vi "Configure Time Tagging.vi"(7 "Virtual Memory Unit in":refnum<class "Virtual Memory Unit.lvclass">, 8 "error in (no error)":errorcluster, 11 "Bus Monitor in":refnum<class "Bus Monitor.lvclass">) -> (0 "error out":errorcluster, 3 "Bus Monitor out":refnum<class "Bus Monitor.lvclass">, 5 "Virtual Memory Unit out":refnum<class "Virtual Memory Unit.lvclass">)   [LabVIEW 2016, in "BCI-1553 API.lvlib" / "Bus Monitor.lvclass"]
uses:
  Bus Monitor.lvclass
  Dependencies/Virtual Memory Unit/Virtual Memory Unit.lvclass
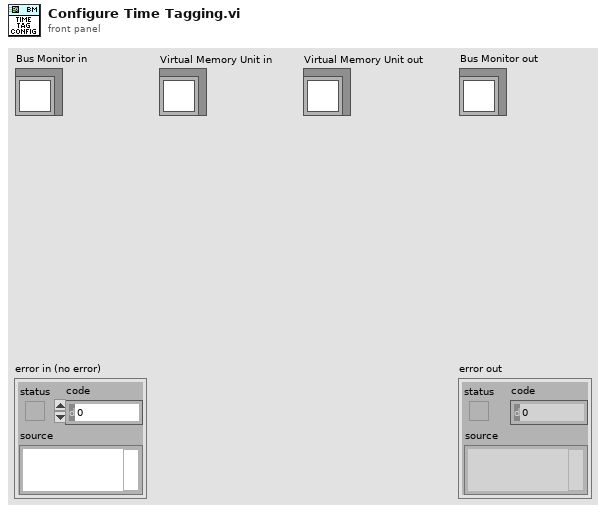
[diagram p1: front panel]
types:
  T1 = typedef "BCI-1553 API.lvlib/Bus Monitor.lvclass/Bus Monitor Timetag Configuration.ctl" = enum16{"Disabled", "2us", "4us", "8us", "16us", "32us", "64us", "100ns"}
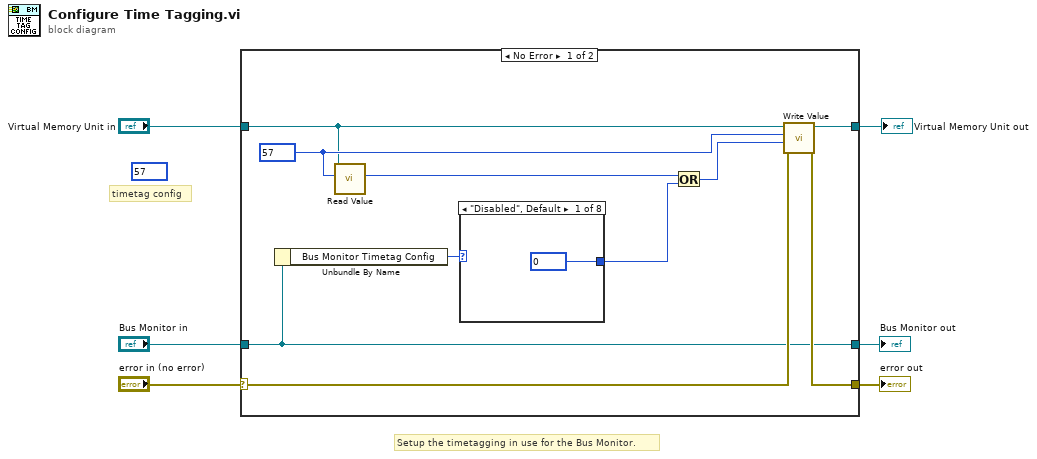
[diagram p0: block diagram]
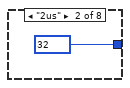
[diagram p2: hidden frame]
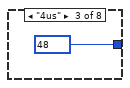
[diagram p3: hidden frame]
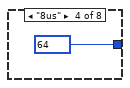
[diagram p4: hidden frame]
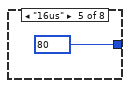
[diagram p5: hidden frame]
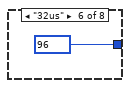
[diagram p6: hidden frame]
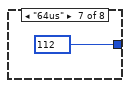
[diagram p7: hidden frame]
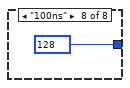
[diagram p8: hidden frame]
diagram:
  (unwired) u16 57 ("Address")
  # "Setup the timetagging in use for the Bus Monitor."
  # "timetag config"
  n1 = case shown="No Error" "error in (no error)" {
    selector: "error in (no error)" -> [w11 w27]
    tunnel: [w10 w27] -> w5
    tunnel: [w9 w26] -> w3
    tunnel: "Bus Monitor in" -> [w9 w26]
    tunnel: "Virtual Memory Unit in" -> [w13 w25]
    tunnel: [w12 w25] -> w1
    frame No Error {
      w16 = 57 ("Address")
      n2 = Unbundle By Name(w9) -> ("Bus Monitor Timetag Config"=w8:T1)
      n3 = call "Read Value.vi"("Index"=w16, "Virtual Memory Unit in"=w13) -> ("Value"=w15:u16)  [unwired: 8 in, 1 out]
      n4 = case shown="\"Disabled\", Default" w8 {
        tunnel: [u16 0 ("Address") u16 32 ("Address") u16 48 ("Address") u16 64 ("Address") u16 80 ("Address") u16 96 ("Address") u16 112 ("Address") u16 128 ("Address")] -> w7
        frame "Disabled", Default {
        }
        frame "2us" {
        }
        frame "4us" {
        }
        frame "8us" {
        }
        frame "16us" {
        }
        frame "32us" {
        }
        frame "64us" {
        }
        frame "100ns" {
        }
      }
      n5 = Or(x=w15, y=w7) -> (x .or. y?=w14:u16)
      n6 = call "Write Value.vi"("error in (no error)"=w11, "Value"=w14, "Index"=w16, "Virtual Memory Unit in"=w13) -> ("error out"=w10:errorcluster, "Virtual Memory Unit out"=w12:refnum<class "Virtual Memory Unit.lvclass">)  [unwired: 6 in]
    }
    frame Error {
    }
  }
  "error out" <- w5
  "Bus Monitor out" <- w3
  "Virtual Memory Unit out" <- w1
